vi "PolyShortBinString.vi"(6 "Units":dbl, 8 "PolyLine":cluster{"X":dbl, "Y":dbl}[](array[cluster]), 9 "Dir":enum16{"CW", "CCW", "Open"}(ring), 10 "ID":u16, 11 "BinStirngIn":string) -> (3 "String":string)   [LabVIEW 2012]
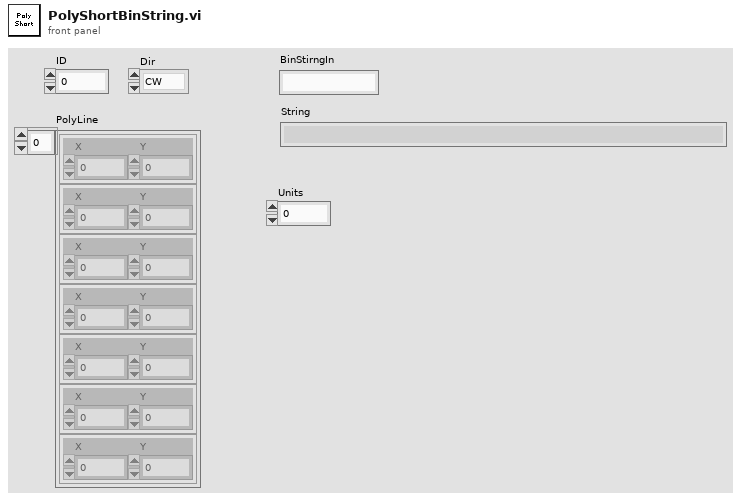
[diagram p1: front panel]
types:
  T1 = enum16{"big-endian, network order", "native, host order", "little-endian"}
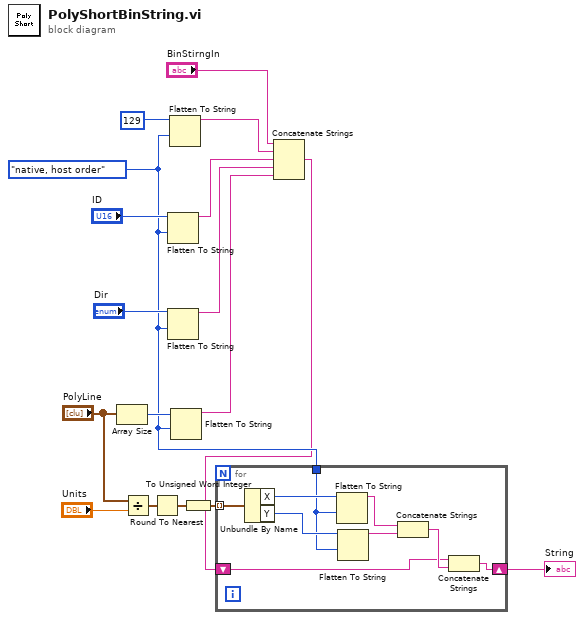
[diagram p0: block diagram]
diagram:
  w10 = T1."native, host order" ("byte order (0:big-endian, network order)")
  n1 = Array Size(array="PolyLine") -> (size(s)=w14:i32)
  n2 = Divide(x="PolyLine", y="Units") -> (x/y=w11:cluster{"X":dbl, "Y":dbl}[])
  n3 = Round To Nearest(number=w11) -> (nearest integer value=w2:cluster{"X":dbl, "Y":dbl}[])
  n4 = Flatten To String(anything="ID", byte order (0:big-endian, network order)=w10) -> (data string=w8:string)  [unwired: 2 in, 2 out]
  n5 = Flatten To String(anything="Dir", byte order (0:big-endian, network order)=w10) -> (data string=w7:string)  [unwired: 2 in, 2 out]
  n6 = Flatten To String(anything=u16 129 ("Layer"), byte order (0:big-endian, network order)=w10) -> (data string=w9:string)  [unwired: 2 in, 2 out]
  n7 = Flatten To String(anything=w14, byte order (0:big-endian, network order)=w10) -> (data string=w6:string)  [unwired: 2 in, 2 out]
  n8 = To Unsigned Word Integer(number=w2) -> (unsigned 16bit integer=w3:cluster{"X":u16, "Y":u16}[])
  n9 = Concatenate Strings("BinStirngIn", w9, w8, w7, w6) -> (w5:string)
  n10 = for {
    tunnel: w3 -> [w26] mode=indexing
    tunnel: w10 -> [w23]
    shift-right: [w18] -> w4
    shift-left: w5 -> [w19]
    n11 = Unbundle By Name(w26) -> ("X"=w25:u16, "Y"=w24:u16)
    n12 = Flatten To String(anything=w25, byte order (0:big-endian, network order)=w23) -> (data string=w22:string)  [unwired: 2 in, 2 out]
    n13 = Flatten To String(anything=w24, byte order (0:big-endian, network order)=w23) -> (data string=w21:string)  [unwired: 2 in, 2 out]
    n14 = Concatenate Strings(w22, w21) -> (w20:string)
    n15 = Concatenate Strings(w19, w20) -> (w18:string)
  }
  "String" <- w4
